vi "Hardware-HHStatus-Host.vi"() -> ()   [LabVIEW 2016]
uses:
  <vilib>/Powertrain Controls/Device Drivers/DCM/HH/RT/Status.ctl
  <vilib>/Powertrain Controls/Device Drivers/DCM/HH/RT/DCM - RT - HH.lvlib
panel:
  out "Status":T1[](array[typedef]) {"Current [A]" format="%#_6p"; "On Avg [A]" format="%#_6p"; "Period Avg [A]" format="%#_6p"; "Period Max [A]" format="%#_6p"; "Period Min [A]" format="%#_6p"}
  out "_Half-H Status":string[][](table) caption="Half-H Status"
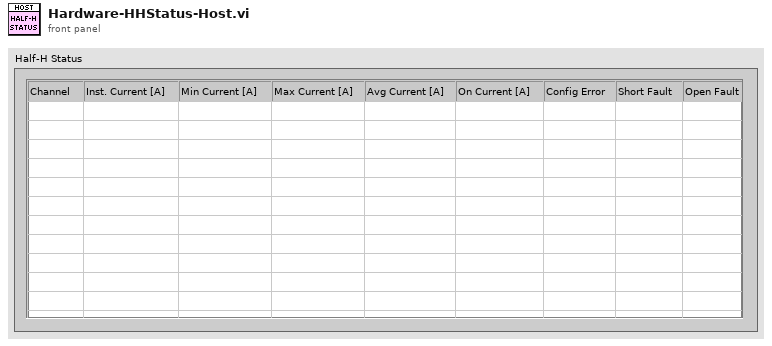
[diagram p1: front panel]
types:
  T1 = typedef "DCM - RT - HH.lvlib/Status.ctl" = cluster{"Current [A]":sgl, "Config Error":bool, "Short Fault":bool, "Open Fault":bool, "Period Min [A]":sgl, "Period Max [A]":sgl, "Period Avg [A]":sgl, "On Avg [A]":sgl}
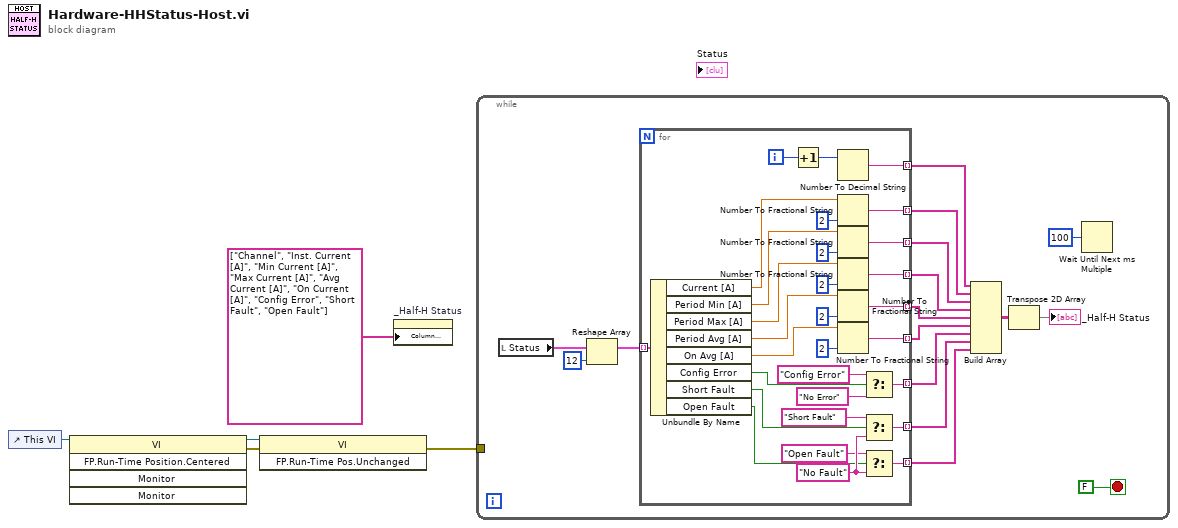
[diagram p0: block diagram]
diagram:
  n1 = control-ref of="This VI"() -> (w2:refnum<vi>)
  n2 = invoke class="VI" method="FP.Run-Time Position.Centered"(reference=w2) -> (reference out=w3:refnum<vi>, error out=w4:errorcluster)  [unwired: 4 in, 3 out]
  n3 = invoke class="VI" method="FP.Run-Time Pos.Unchanged"(reference=w3, error in=w4) -> (error out=w1:errorcluster)  [unwired: 1 in, 2 out]
  n4 = property on="_Half-H Status" class="Tbl (strict)"("Column Headers[]"=string[] ["Channel", "Inst. Current [A]", "Min Current [A]", "Max Current [A]", "Avg Current [A]", "On Current [A]", "Config Error", "Short Fault", "Open Fault"] ("Column Header Strings[]")) -> ()  [unwired: 2 in, 2 out]
  n5 = while {
    tunnel: w1 -> [_]
    stop <- FALSE stop-if-true
    n6 = local read "Status"() -> (w6:T1[])
    n7 = Reshape Array(w6, 12 ("dimension size")) -> (w12:T1[])
    n8 = for {
      tunnel: w12 -> [w51] mode=indexing
      tunnel: [w40] -> w18 mode=indexing
      tunnel: [w39] -> w17 mode=indexing
      tunnel: [w38] -> w16 mode=indexing
      tunnel: [w37] -> w15 mode=indexing
      tunnel: [w32] -> w8 mode=indexing
      tunnel: [w31] -> w7 mode=indexing
      tunnel: [w29] -> w9 mode=indexing
      tunnel: [w28] -> w19 mode=indexing
      tunnel: [w25] -> w10 mode=indexing
      i -> [w27]
      w34 = "No Fault"
      n9 = Unbundle By Name(w51) -> ("Current [A]"=w50:sgl, "Period Min [A]"=w44:sgl, "Period Max [A]"=w43:sgl, "Period Avg [A]"=w42:sgl, "On Avg [A]"=w41:sgl, "Config Error"=w24:bool, "Short Fault"=w23:bool, "Open Fault"=w22:bool)
      n10 = Increment(x=w27) -> (x+1=w26:i32)
      n11 = Number To Decimal String(number=w26) -> (decimal integer string=w25:string)  [unwired: 1 in]
      n12 = Number To Fractional String(number=w50, precision (6)=i16 2) -> (F-format string=w28:string)  [unwired: 2 in]
      n13 = Number To Fractional String(number=w44, precision (6)=i16 2) -> (F-format string=w40:string)  [unwired: 2 in]
      n14 = Number To Fractional String(number=w43, precision (6)=i16 2) -> (F-format string=w39:string)  [unwired: 2 in]
      n15 = Number To Fractional String(number=w42, precision (6)=i16 2) -> (F-format string=w38:string)  [unwired: 2 in]
      n16 = Number To Fractional String(number=w41, precision (6)=i16 2) -> (F-format string=w37:string)  [unwired: 2 in]
      n17 = Select(t="Config Error", s=w24, f="No Error") -> (s? t:f=w29:string)
      n18 = Select(t="Short Fault", s=w23, f=w34) -> (s? t:f=w32:string)
      n19 = Select(t="Open Fault", s=w22, f=w34) -> (s? t:f=w31:string)
    }
    n20 = Build Array(w10, w19, w18, w17, w16, w15, w9, w8, w7) -> (w14:string[][])
    n21 = Transpose 2D Array(2D array=w14) -> (transposed array=→"_Half-H Status":string[][])
    n22 = Wait Until Next ms Multiple(millisecond multiple=u32 100) -> ()  [unwired: 1 out]
  }
